vi "Test Motor API.vi"() -> ()   [LabVIEW 2022 SP3]
doc: "Motor API Tester."
uses:
  <vilib>/Utility/error.llb/DialogType.ctl
  Motor.lvlib
panel:
  out "last error":errorcluster
  in  "Show Diagram on Init":bool
  in  "Show Block Diagram":bool
  in  "Stop Module":bool
  in  "Start Module":bool
  in  "Hide Module Panel":bool
  in  "Show Module Panel":bool
  out "Status":string
  out "Module Running?":bool
  # "This VI tests the API for the Module."
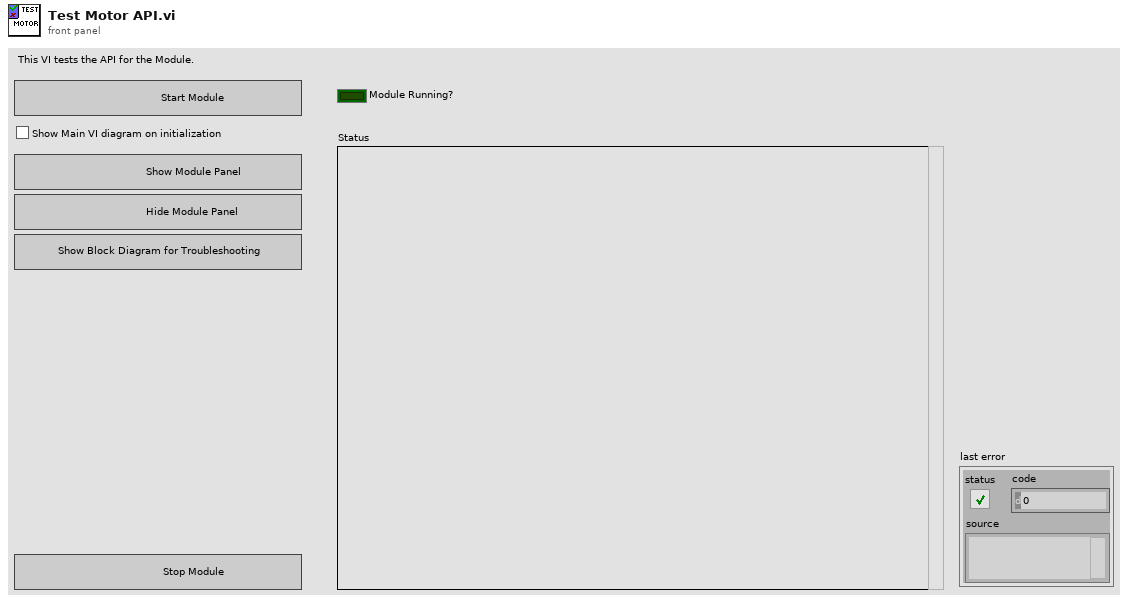
[diagram p1: front panel]
types:
  T1 = typedef "Motor.lvlib/Broadcast Events--cluster.ctl" = cluster{"Module Did Init":refnum<user-event>, "Status Updated":refnum<user-event>, "Error Reported":refnum<user-event>, "Did Something":refnum<user-event>, "Module Did Stop":refnum<user-event>, "Update Module Execution Status":refnum<user-event>}
  T2 = typedef "DialogType.ctl" = u16
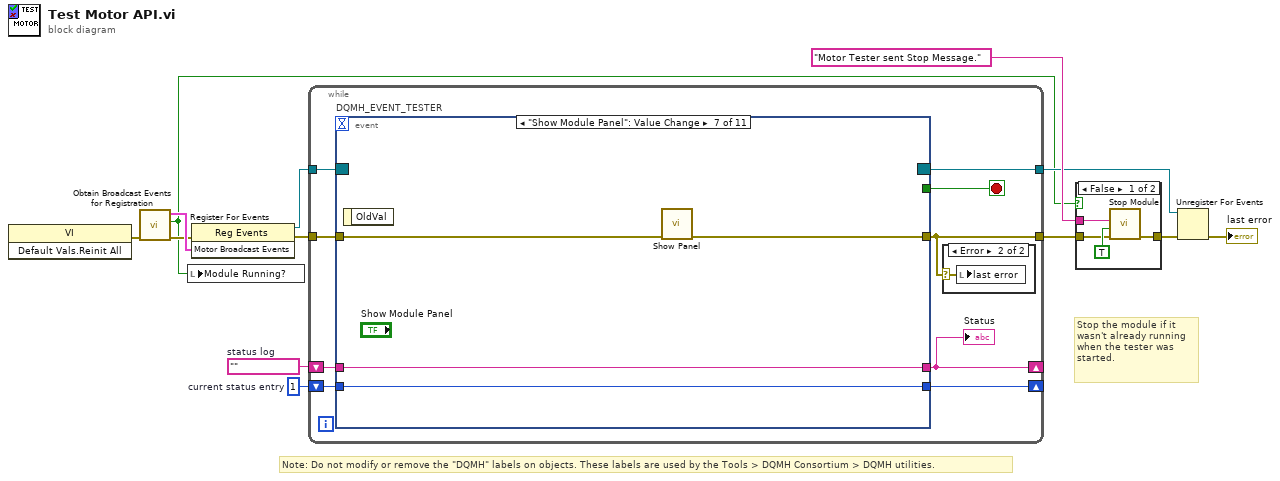
[diagram p0: block diagram]
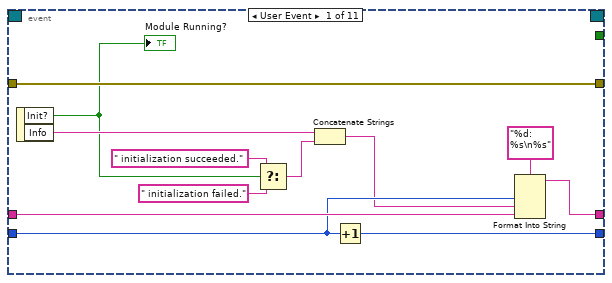
[diagram p4: hidden frame]
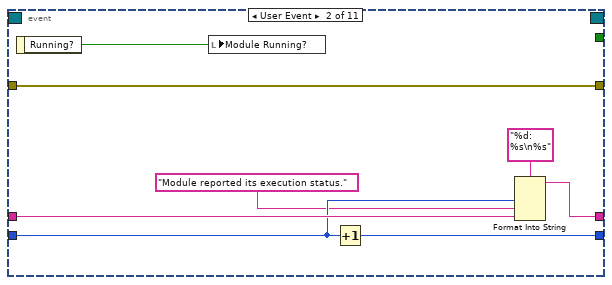
[diagram p5: hidden frame]
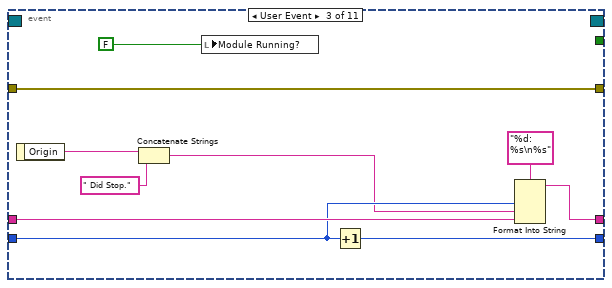
[diagram p6: hidden frame]
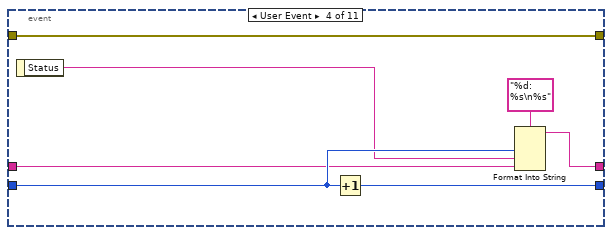
[diagram p7: hidden frame]
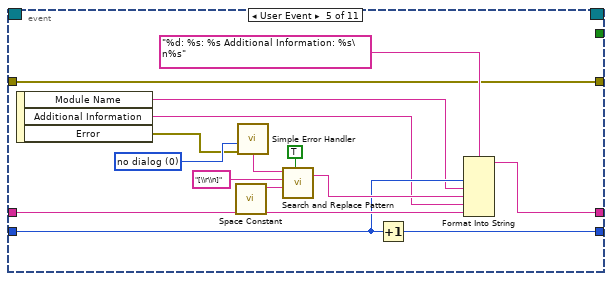
[diagram p8: hidden frame]
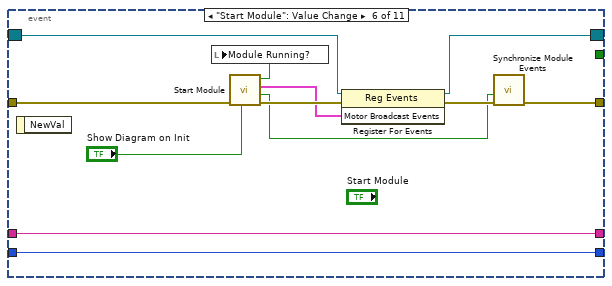
[diagram p9: hidden frame]
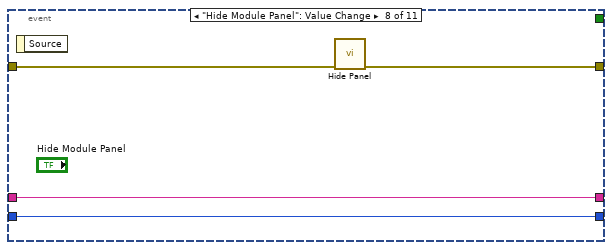
[diagram p10: hidden frame]
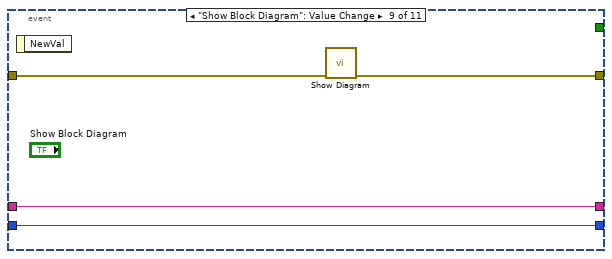
[diagram p11: hidden frame]
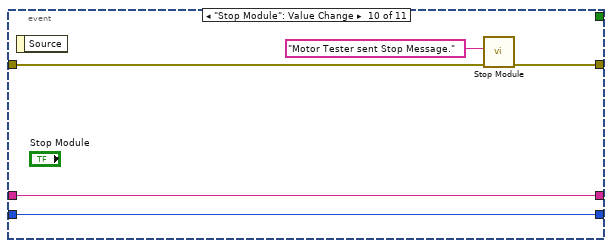
[diagram p12: hidden frame]
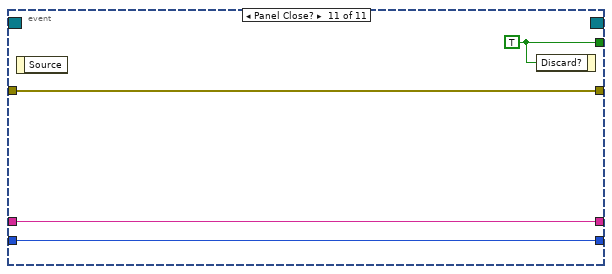
[diagram p13: hidden frame]
diagram:
  w10 = 1  # current status entry
  w11 = ""  # status log
  # "Stop the module if it wasn't already running when the tester was started."
  # "Note: Do not modify or remove the \"DQMH\" labels on objects. These labels are used by the Tools > DQMH Consortium > DQMH utilities."
  n1 = invoke class="VI" method="Default Vals.Reinit All"() -> (error out=w5:errorcluster)  [unwired: 3 in, 2 out]
  n2 = call "Obtain Broadcast Events for Registration.vi"("error in"=w5) -> ("error out"=w4:errorcluster, "Already running?"=w3:bool, "Motor Broadcast Events"=w8:T1)  [unwired: 8 in]
  n3 = local write "Module Running?"(w3) -> ()
  n4 = register-events(error in=w4, w8) -> (reference out=w7:refnum<event-registration>, error out=w9:errorcluster)  [unwired: 1 in]
  n5 = while {
    tunnel: w7 -> [w22]
    tunnel: [w14] -> w2
    shift-right: [w18] -> _
    shift-left: w11 -> [w20]
    shift-right: [w19] -> _
    shift-left: w10 -> [w21]
    tunnel: w9 -> [w17]
    tunnel: [w16] -> w6
    stop <- w15 stop-if-true
    n6 = event "DQMH_EVENT_TESTER" shown="[6] \"Show Module Panel\": Value Change" {
      selector: w22 -> [_ _ _ _ _ w81 _ _ _ _ _]
      dyn-events: [_ _ _ _ _ w80 _ _ _ _ _] -> w16
      timeout: _ -> [_ _ _ _ _ _ _ _ _ _ _]
      tunnel: [_ _ _ _ _ _ _ _ _ _ w108] -> w15
      tunnel: [w35 w37 w44 w54 w64 w79 w91 w95 w96 w102 w105] -> w14
      tunnel: w21 -> [w32 w41 w51 w57 w67 w84 w89 w93 w97 w103 w106]
      tunnel: w20 -> [w33 w42 w52 w56 w68 w85 w90 w94 w98 w104 w107]
      tunnel: [w30 w39 w49 w58 w66 w85 w90 w94 w98 w104 w107] -> w18
      tunnel: [w31 w40 w50 w60 w65 w84 w89 w93 w97 w103 w106] -> w19
      tunnel: w17 -> [w35 w37 w44 w54 w64 w78 w88 w92 w99 w100 w105]
      event User Event {
        n7 = event-data() -> ("Init?"=w27:bool, "Info"=w29:string)  [unwired: 1 in]
        "Module Running?" <- w27
        n8 = Select(t=" initialization succeeded.", s=w27, f=" initialization failed.") -> (s? t:f=w24:string)
        n9 = Concatenate Strings(w29, w24) -> (w28:string)
        n10 = Increment(x=w32) -> (x+1=w31:i32)
        n11 = Format Into String(format string="%d: %s\n%s", w32, w28, w33) -> (resulting string=w30:string)  [unwired: 2 in, 1 out]
      }
      event User Event {
        n12 = event-data() -> ("Running?"=w36:bool)  [unwired: 1 in]
        n13 = local write "Module Running?"(w36) -> ()
        n14 = Increment(x=w41) -> (x+1=w40:i32)
        n15 = Format Into String(format string="%d: %s\n%s", w41, "Module reported its execution status.", w42) -> (resulting string=w39:string)  [unwired: 2 in, 1 out]
      }
      event User Event {
        n16 = event-data() -> ("Origin"=w48:string)  [unwired: 1 in]
        n17 = Concatenate Strings(w48, " Did Stop.") -> (w47:string)
        n18 = local write "Module Running?"(FALSE ("Module Did Init?")) -> ()
        n19 = Increment(x=w51) -> (x+1=w50:i32)
        n20 = Format Into String(format string="%d: %s\n%s", w51, w47, w52) -> (resulting string=w49:string)  [unwired: 2 in, 1 out]
      }
      event User Event {
        n21 = event-data() -> ("Status"=w55:string)  [unwired: 1 in]
        n22 = Increment(x=w57) -> (x+1=w60:i32)
        n23 = Format Into String(format string="%d: %s\n%s", w57, w55, w56) -> (resulting string=w58:string)  [unwired: 2 in, 1 out]
      }
      event User Event {
        w69 = T2 0 items=["no dialog", "OK message", "continue or stop message", "OK message + warnings", "continue/stop + warnings"] ("type of dialog (OK msg:1)")
        n24 = event-data() -> ("Module Name"=w63:string, "Additional Information"=w62:string, "Error"=w61:errorcluster)  [unwired: 1 in]
        n25 = call <vilib>:"Space Constant.vi"() -> ("String"=w73:string)
        n26 = call <vilib>:"Simple Error Handler.vi"("type of dialog (OK msg:1)"=w69, "error in (no error)"=w61) -> ("message"=w70:string)  [unwired: 3 in, 4 out]
        n27 = call <vilib>:"Search and Replace Pattern.vi"("string"=w70, "regular expression (\"\")"="[\\r\\n]" ("regular expression (\"\")"), "replace string (\"\")"=w73, "replace all? (F)"=TRUE ("replace all CR/LF with spaces")) -> ("result string"=w71:string)  [unwired: 1 in, 1 out]
        n28 = Increment(x=w67) -> (x+1=w65:i32)
        n29 = Format Into String(format string="%d: %s: %s Additional Information: %s\n%s", w67, w63, w71, w62, w68) -> (resulting string=w66:string)  [unwired: 2 in, 1 out]
      }
      event "Start Module": Value Change {
        n30 = event-data() -> ()  [unwired: 1 in, 1 out]
        n31 = call "Start Module.vi"("Show Main VI Diagram on Init (F)"="Show Diagram on Init", "error in"=w78) -> ("error out"=w86:errorcluster, "Wait for Event Sync?"=w83:bool, "Motor Broadcast Events"=w82:T1, "Module Was Already Running?"=w77:bool)  [unwired: 6 in]
        n32 = local write "Module Running?"(w77) -> ()
        n33 = register-events(reference=w81, error in=w86, w82) -> (reference out=w80:refnum<event-registration>, error out=w87:errorcluster)
        n34 = call "Synchronize Module Events.vi"("error in"=w87, "Wait for Event Sync?"=w83) -> ("error out"=w79:errorcluster)  [unwired: 9 in]
      }
      event "Show Module Panel": Value Change {
        n35 = event-data() -> ()  [unwired: 1 in, 1 out]
        n36 = call "Show Panel.vi"("error in"=w88) -> ("error out"=w91:errorcluster)  [unwired: 10 in]
      }
      event "Hide Module Panel": Value Change {
        n37 = event-data() -> ()  [unwired: 1 in, 1 out]
        n38 = call "Hide Panel.vi"("error in"=w92) -> ("error out"=w95:errorcluster)  [unwired: 10 in]
      }
      event "Show Block Diagram": Value Change {
        n39 = event-data() -> ()  [unwired: 1 in, 1 out]
        n40 = call "Show Diagram.vi"("error in"=w99) -> ("error out"=w96:errorcluster)  [unwired: 10 in]
      }
      event "Stop Module": Value Change {
        n41 = event-data() -> ()  [unwired: 1 in, 1 out]
        n42 = call "Stop Module.vi"("error in"=w100, "Origin"="Motor Tester sent Stop Message.") -> ("error out"=w102:errorcluster)  [unwired: 9 in]
      }
      event Panel Close? {
        w108 = TRUE ("Discard?")
        n43 = event-data() -> ()  [unwired: 1 in, 1 out]
        n44 = event-data("Discard?"=w108) -> ()  [unwired: 1 in, 1 out]
      }
    }
    "Status" <- w18
    n45 = case shown="Error" w14 {
      selector: w14 -> [_ w23]
      frame No Error {
      }
      frame Error {
        n46 = local write "last error"(w23) -> ()
      }
    }
  }
  n47 = case shown="False" w3 {
    tunnel: [w112 w113] -> w13
    tunnel: "Motor Tester sent Stop Message." ("Origin") -> [w111 _]
    tunnel: w2 -> [w109 w113]
    frame False {
      n48 = call "Stop Module.vi"("error in"=w109, "Wait for Module to Stop? (F)"=TRUE ("Wait for Module to stop?"), "Origin"=w111) -> ("error out"=w112:errorcluster)  [unwired: 8 in]
    }
    frame True {
    }
  }
  n49 = Unregister For Events(event registration refnum=w6, error in=w13) -> (error out=→"last error":errorcluster)
